vi "QueryUSNO.vi"(5 "wget":path, 7 "Data dir Path":path, 8 "mag_limit":dbl, 9 "radius":dbl, 10 "DEC":dbl format="%.6g", 11 "RA":dbl format="%.6g") -> (0 "Data OUT":string[][](array[string]), 3 "Data File Path":path, 4 "No Error":bool)   [LabVIEW 2011]
uses:
  <vilib>/Utility/file.llb/Read From Spreadsheet File (string).vi
  <vilib>/Utility/file.llb/Write To Spreadsheet File (string).vi
panel:
  out "error out":errorcluster
  out "CMD Error":errorcluster
  out "rm Error":errorcluster[](array[cluster])
  out "Complete command ...":string
  out "standard error":string
  out "standard output":string
  out "identifier":string
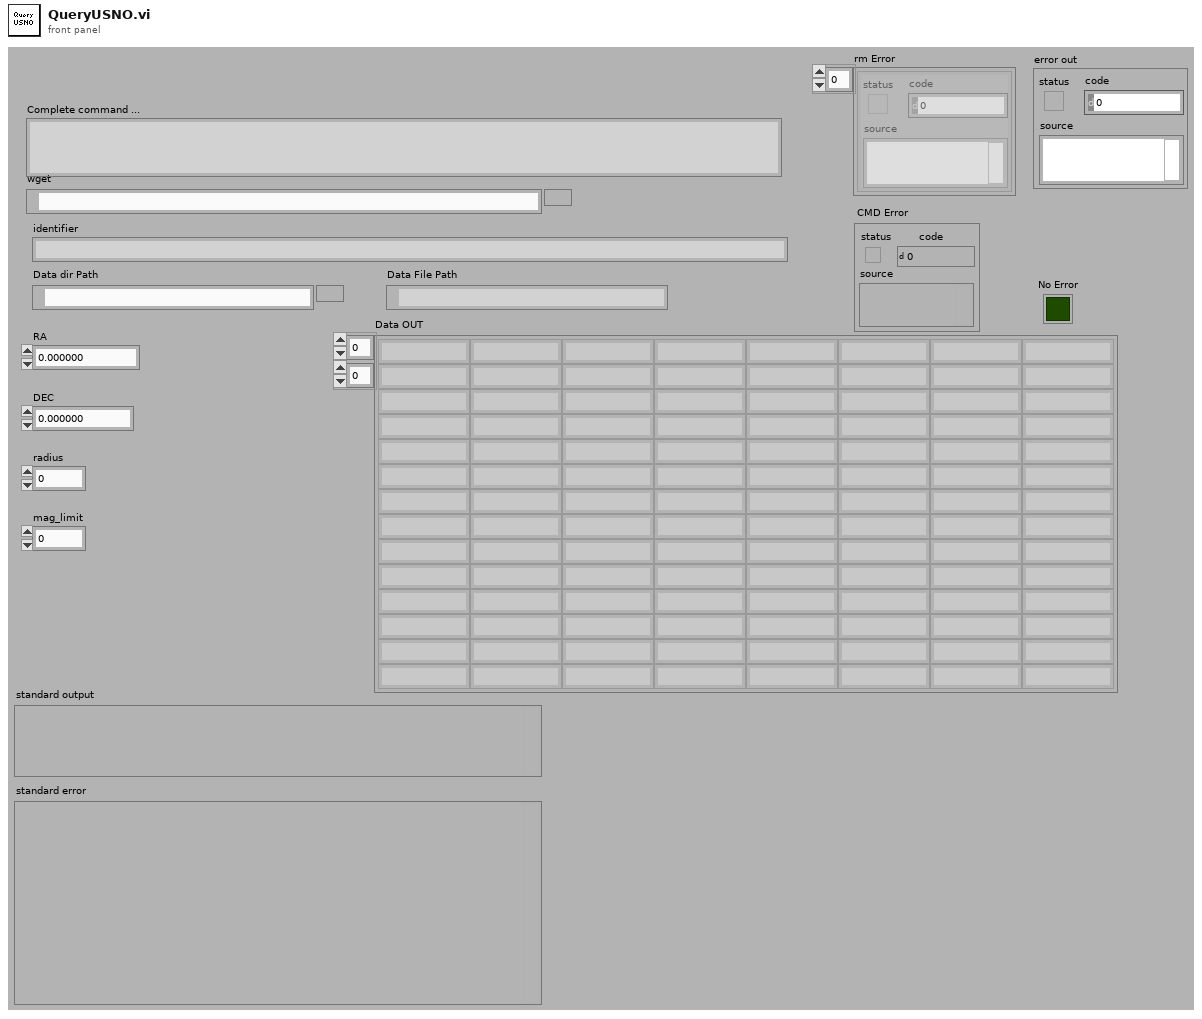
[diagram p1: front panel]
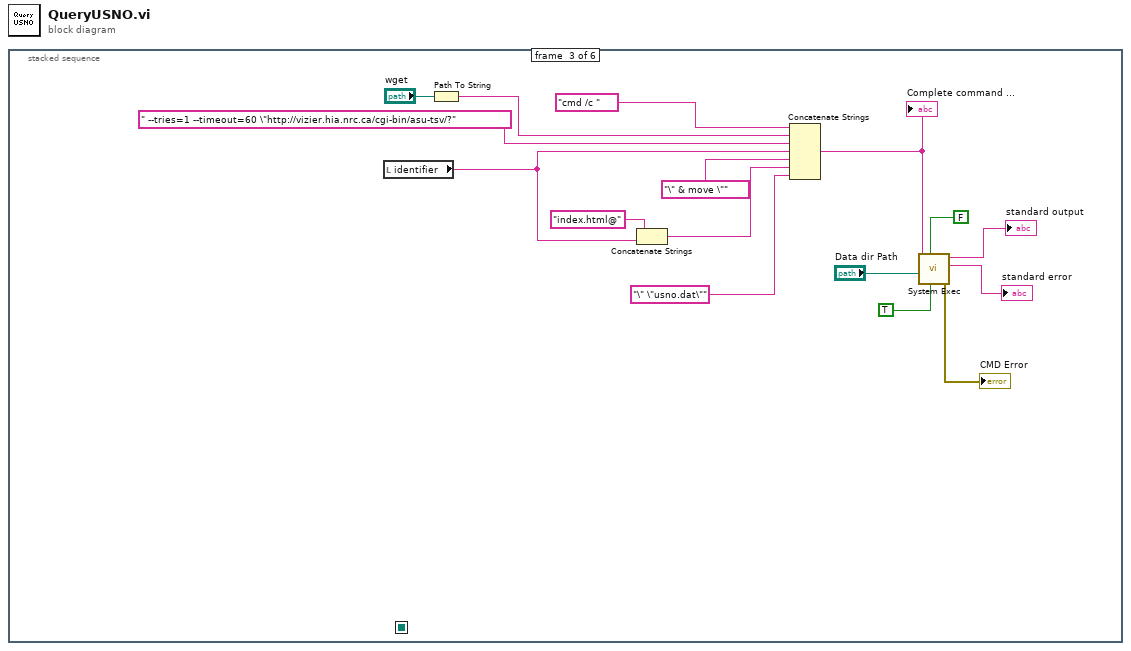
[diagram p0: block diagram]
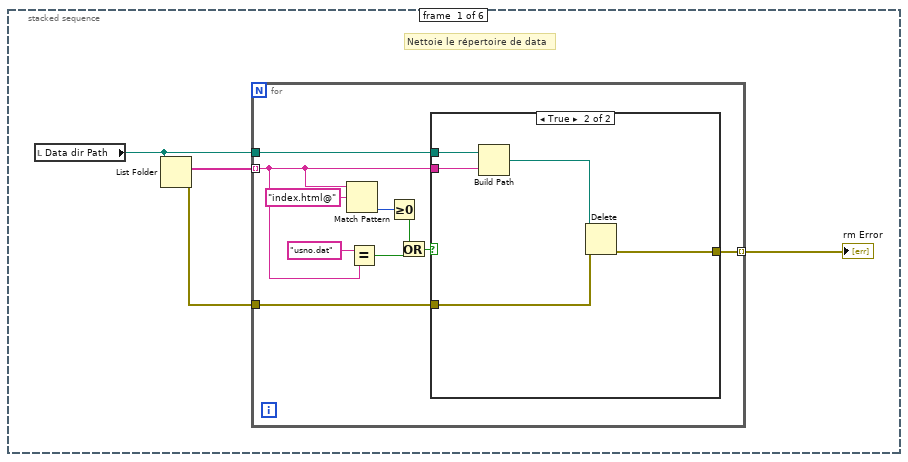
[diagram p2: hidden frame]
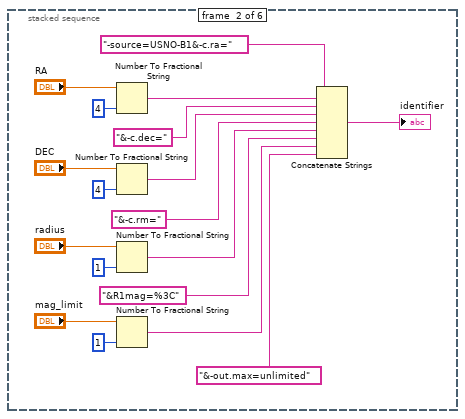
[diagram p4: hidden frame]
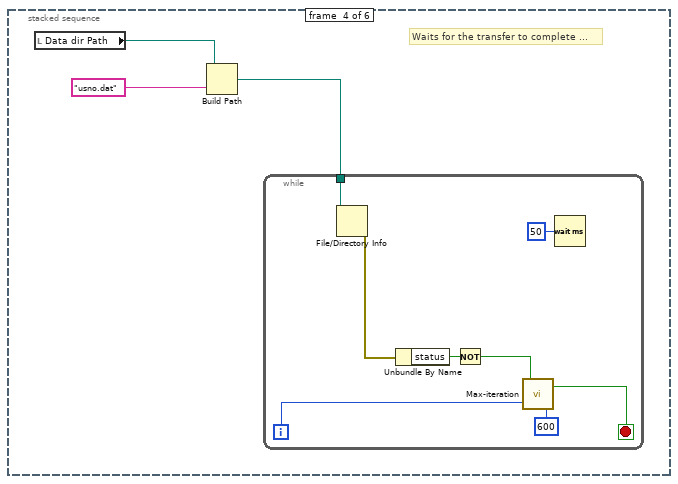
[diagram p5: hidden frame]
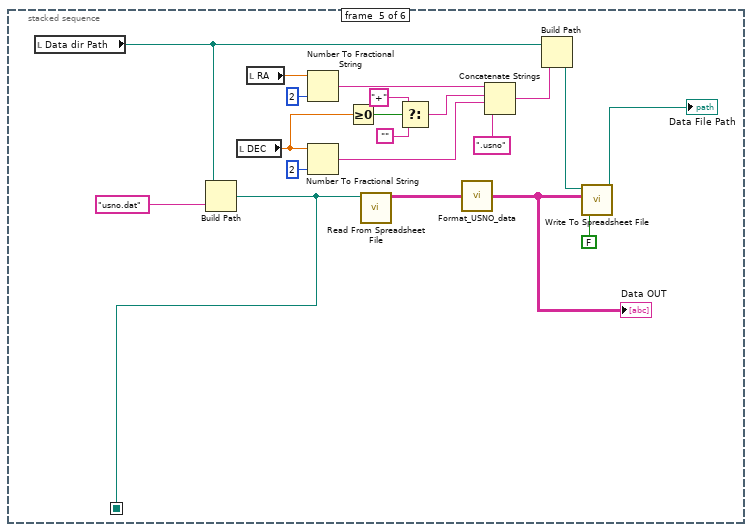
[diagram p6: hidden frame]
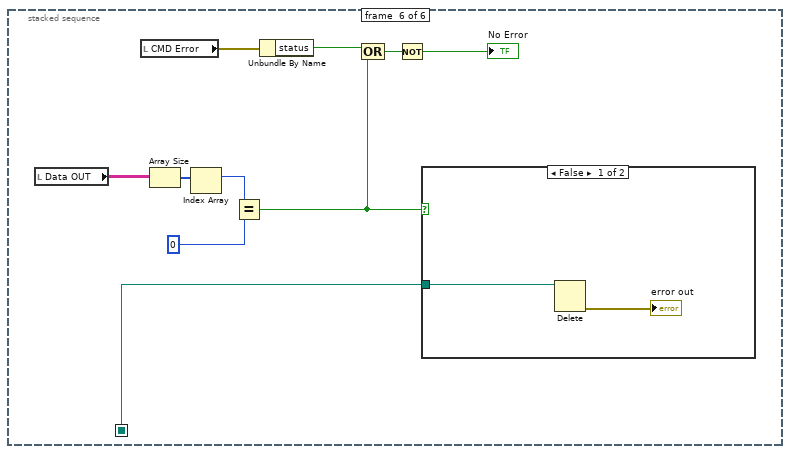
[diagram p7: hidden frame]
diagram:
  n1 = stacked-sequence {
    seq-local: [_ _ _ _ w85 _] -> [_ _ _ _ _ w86]
    frame #0 {
      # "Nettoie le répertoire de data"
      n2 = local read "Data dir Path"() -> (w3:path)
      n3 = List Folder(path=w3) -> (filenames=w4:string[], error out=w2:errorcluster)  [unwired: 3 in, 2 out]
      n4 = for {
        tunnel: w4 -> [w5] mode=indexing
        tunnel: w3 -> [w14]
        tunnel: w2 -> [w11]
        tunnel: [w10] -> w1 mode=indexing
        n5 = Match Pattern(string=w5, regular expression="index.html@") -> (offset past match=w12:i32)  [unwired: 1 in, 3 out]
        n6 = Equal?(x="usno.dat" ("regular expression"), y=w5) -> (x = y?=w6:bool)
        n7 = Greater Or Equal To 0?(x=w12) -> (x >= 0?=w8:bool)
        n8 = Or(x=w8, y=w6) -> (x .or. y?=w9:bool)
        n9 = case shown="True" w9 {
          tunnel: w5 -> [_ w20]
          tunnel: w14 -> [_ w19]
          tunnel: w11 -> [w15 w17]
          tunnel: [w15 w16] -> w10
          frame False {
          }
          frame True {
            n10 = Build Path(base path=w19, name or relative path=w20) -> (appended path=w18:path)
            n11 = Delete(path (use dialog)=w18, error in=w17) -> (error out=w16:errorcluster)  [unwired: 3 in, 2 out]
          }
        }
      }
      "rm Error" <- w1
    }
    frame #1 {
      n12 = Number To Fractional String(number="RA", precision (6)=i16 4) -> (F-format string=w36:string)  [unwired: 2 in]
      n13 = Number To Fractional String(number="DEC", precision (6)=i16 4) -> (F-format string=w30:string)  [unwired: 2 in]
      n14 = Number To Fractional String(number="radius", precision (6)=i16 1) -> (F-format string=w28:string)  [unwired: 2 in]
      n15 = Number To Fractional String(number="mag_limit", precision (6)=i16 1) -> (F-format string=w24:string)  [unwired: 2 in]
      n16 = Concatenate Strings("-source=USNO-B1&-c.ra=", w36, "&-c.dec=", w30, "&-c.rm=", w28, "&R1mag=%3C", w24, "&-out.max=unlimited") -> (→"identifier":string)
    }
    frame #2 {
      n17 = local read "identifier"() -> (w40:string)
      n18 = Path To String(path="wget") -> (string=w47:string)
      n19 = Concatenate Strings("index.html@", w40) -> (w39:string)
      n20 = Concatenate Strings("cmd /c " ("string"), w47, " --tries=1 --timeout=60 \"http://vizier.hia.nrc.ca/cgi-bin/asu-tsv/?", w40, "\" & move \"", w39, "\" \"usno.dat\"" ("string")) -> (w53:string)
      "Complete command ..." <- w53
      n21 = call <vilib>:"System Exec.vi"("run minimized? (F)"=TRUE, "wait until completion? (T)"=FALSE, "working directory"="Data dir Path", "command line"=w53) -> ("error out"=→"CMD Error":errorcluster, "standard error"=→"standard error":string, "standard output"=→"standard output":string)  [unwired: 4 in, 1 out]
    }
    frame #3 {
      # "Waits for the transfer to complete ..."
      n22 = local read "Data dir Path"() -> (w57:path)
      n23 = Build Path(base path=w57, name or relative path="usno.dat") -> (appended path=w56:path)
      n24 = while {
        tunnel: w56 -> [w65]
        i -> [w63]
        stop <- w61 stop-if-true
        n25 = File/Directory Info(path=w65) -> (error out=w59:errorcluster)  [unwired: 1 in, 6 out]
        n26 = Unbundle By Name(w59) -> ("status"=w58:bool)
        n27 = Not(x=w58) -> (.not. x?=w60:bool)
        n28 = call "Max-iteration.vi"("i max"=600, "i act"=w63, "Valeur entrante"=w60) -> ("break ?"=w61:bool)
        n29 = Wait (ms)(milliseconds to wait=u32 50) -> ()  [unwired: 1 out]
      }
    }
    frame #4 {
      n30 = local read "Data dir Path"() -> (w82:path)
      n31 = Build Path(base path=w82, name or relative path="usno.dat") -> (appended path=w85:path)
      n32 = local read "DEC"() -> (w75:dbl)
      n33 = local read "RA"() -> (w78:dbl)
      n34 = Number To Fractional String(number=w78, precision (6)=i16 2) -> (F-format string=w73:string)  [unwired: 2 in]
      n35 = Number To Fractional String(number=w75, precision (6)=i16 2) -> (F-format string=w69:string)  [unwired: 2 in]
      n36 = Greater Or Equal To 0?(x=w75) -> (x >= 0?=w74:bool)
      n37 = call-poly <vilib>:"Read From Spreadsheet File.vi"("file path (dialog if empty)"=w85) -> ("all rows"=w84:string[][])  [unwired: 6 in, 4 out]
      n38 = Select(t="+", s=w74, f="") -> (s? t:f=w72:string)
      n39 = call "Format_USNO_data.vi"("Data IN"=w84) -> ("Data OUT"=w83:string[][])  [unwired: 4 in]
      "Data OUT" <- w83
      n40 = Concatenate Strings(w73, w72, w69, ".usno" ("string")) -> (w67:string)
      n41 = Build Path(base path=w82, name or relative path=w67) -> (appended path=w81:path)
      n42 = call-poly <vilib>:"Write To Spreadsheet File.vi"("append to file? (new file:F)"=FALSE, "2D data"=w83, "file path (dialog if empty)"=w81) -> ("new file path (Not A Path if cancelled)"=→"Data File Path":path)  [unwired: 5 in]
    }
    frame #5 {
      n43 = local read "Data OUT"() -> (w95:string[][])
      n44 = local read "CMD Error"() -> (w93:errorcluster)
      n45 = Array Size(array=w95) -> (size(s)=w94:i32[])
      n46 = Index Array(array=w94) -> (element=w91:i32)  [unwired: 1 in]
      n47 = Equal?(x=w91, y=0) -> (x = y?=w87:bool)
      n48 = Unbundle By Name(w93) -> ("status"=w92:bool)
      n49 = Compound Arithmetic op=OR(w92, w87) -> (w89:bool)
      n50 = Not(x=w89) -> (.not. x?=→"No Error":bool)
      n51 = case shown="False" w87 {
        tunnel: w86 -> [w97 _]
        frame False {
          n52 = Delete(path (use dialog)=w97) -> (error out=→"error out":errorcluster)  [unwired: 4 in, 2 out]
        }
        frame True {
        }
      }
    }
  }
